vi "Test Build TS Activation Execution Plan.vi"() -> (0 "error out":errorcluster)   [LabVIEW 2025]
doc: "This VI tests the logic for building execution plans to activate TestStand versions."
uses:
  src/TSDiscovery Mock/TSDiscovery Mock.lvclass
  <vilib>/addons/_JKI Toolkits/Caraya/classes/Test/Test.lvclass
  <vilib>/addons/_JKI Toolkits/Caraya/classes/Assert/Assert.lvclass
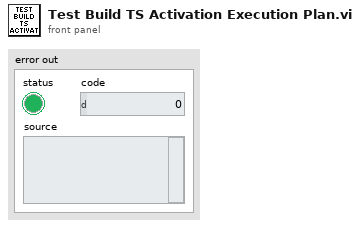
[diagram p1: front panel]
types:
  T1 = typedef "TSInstall--cluster.ctl" = cluster{"Version":string, "Architecture":T2, "Version Key":string, "ID":string}
  T2 = typedef "Architecture--enum.ctl" = enum16{"32bit", "64bit"}
  T3 = typedef "Execution Plan--cluster.ctl" = cluster{"Exe Path":path, "Args":string[], "Timeout":i32}
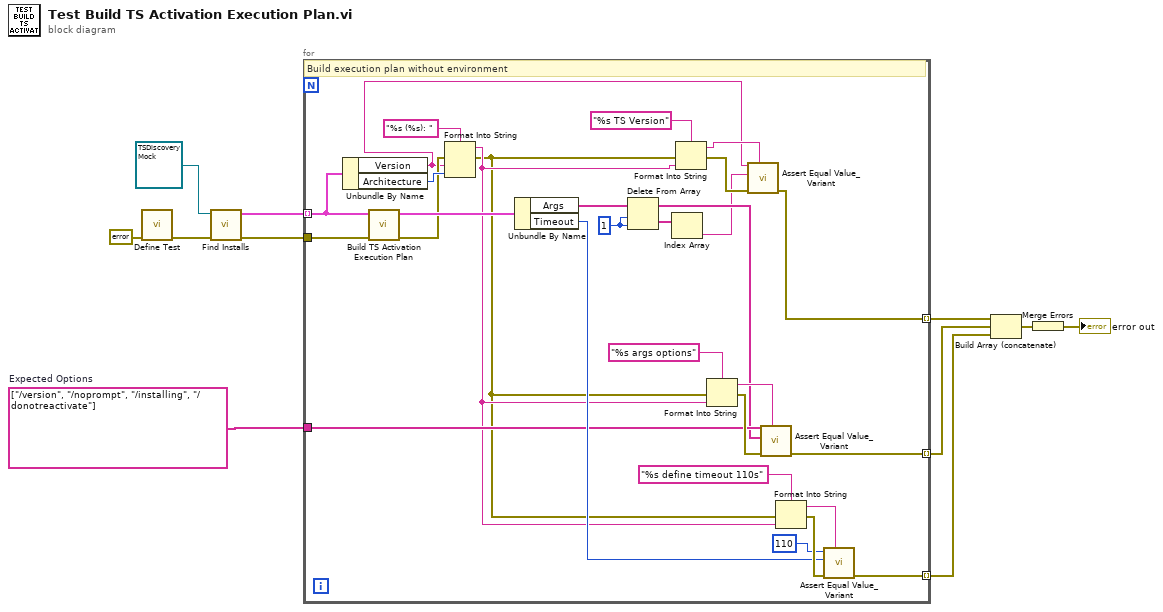
[diagram p0: block diagram]
diagram:
  w2 = string[] ["/version", "/noprompt", "/installing", "/donotreactivate"]  # Expected Options
  n1 = call <vilib>:"Define Test.vi"("error in (no error)"=errorcluster {"status"=FALSE, "code"=0, "source"=""}) -> ("error out"=w10:errorcluster)  [unwired: 9 in, 1 out]
  n2 = call-dynamic "Find Installs.vi"("error in"=w10, "TSDiscovery Mock in"=refnum<class "TSDiscovery Mock.lvclass"> refnum) -> ("error out"=w5:errorcluster, "TSInstalls Out"=w6:T1[])  [unwired: 8 in]
  n3 = for {
    tunnel: w6 -> [w40] mode=indexing
    tunnel: [w27] -> w8 mode=indexing
    tunnel: [w26] -> w7 mode=indexing
    tunnel: w5 -> [w37]
    tunnel: w2 -> [w25]
    tunnel: [w14] -> w1 mode=indexing
    w23 = 1 ("index")
    # "Build execution plan without environment"
    n4 = Unbundle By Name(w40) -> ("Version"=w16:string, "Architecture"=w38:T2)
    n5 = call "Build TS Activation Execution Plan.vi"("error in"=w37, "TSInstall"=w40) -> ("error out"=w31:errorcluster, "Execution Plan"=w36:T3)  [unwired: 8 in]
    n6 = Format Into String(format string="%s (%s): ", error in=w31, w16, w38) -> (resulting string=w19:string, error out=w13:errorcluster)  [unwired: 1 in]
    n7 = Unbundle By Name(w36) -> ("Args"=w24:string[], "Timeout"=w29:i32)
    n8 = Delete From Array(array=w24, length=w23, index=w23) -> (deleted portion=w21:string[], array with subset deleted=w22:string[])
    n9 = Index Array(array=w21) -> (element=w15:string)  [unwired: 1 in]
    n10 = Format Into String(format string="%s TS Version", error in=w13, w19) -> (resulting string=w18:string, error out=w17:errorcluster)  [unwired: 1 in]
    n11 = Format Into String(format string="%s args options", error in=w13, w19) -> (resulting string=w33:string, error out=w34:errorcluster)  [unwired: 1 in]
    n12 = call <vilib>:"Assert Equal Value_Variant.vi"("Label"=w18, "error in (no error)"=w17, "Actual"=w15, "Expected"=w16) -> ("error out"=w14:errorcluster)  [unwired: 6 in, 1 out]
    n13 = call <vilib>:"Assert Equal Value_Variant.vi"("Label"=w33, "error in (no error)"=w34, "Actual"=w22, "Expected"=w25) -> ("error out"=w27:errorcluster)  [unwired: 6 in, 1 out]
    n14 = Format Into String(format string="%s define timeout 110s", error in=w13, w19) -> (resulting string=w12:string, error out=w30:errorcluster)  [unwired: 1 in]
    n15 = call <vilib>:"Assert Equal Value_Variant.vi"("Label"=w12, "error in (no error)"=w30, "Actual"=w29, "Expected"=110) -> ("error out"=w26:errorcluster)  [unwired: 6 in, 1 out]
  }
  n16 = Build Array (concatenate)(w1, w8, w7) -> (w4:errorcluster[])
  n17 = Merge Errors(w4) -> (→"error out":errorcluster)
